vi "TesterOption (SubVI).vi"(8 "error in (no error)":errorcluster, 9 "On/Off":bool=TRUE, 10 "Tester Option":T1(ring), 11 "VISA Refnum in":refnum<visa-resource-name>) -> (0 "error out":errorcluster, 3 "VISA Refnum out":refnum<visa-resource-name>)   [LabVIEW 2017]
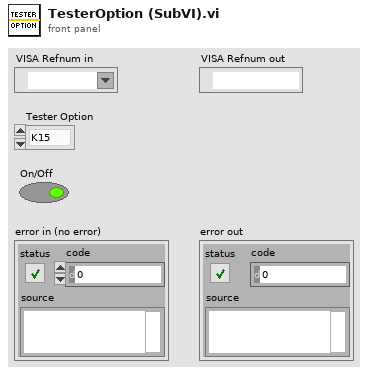
[diagram p1: front panel]
types:
  T1 = enum16{"K15", "K16", "K17", "Venable", "Firmeware", "Fan", "Power", "120C", "110C", "100C", "90C", "80C", "70C", "60C", "50C", "40C", "30C", "25C", "20C", "10C", "0C"}
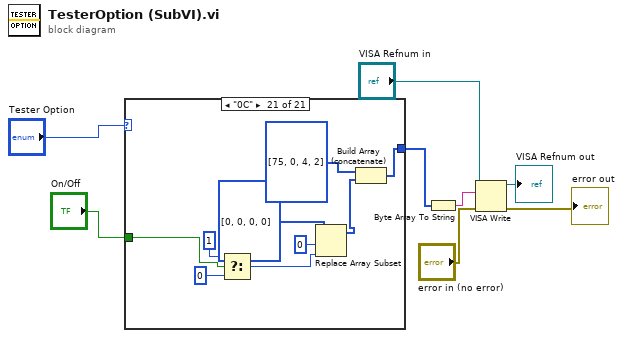
[diagram p0: block diagram]
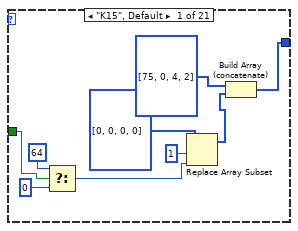
[diagram p2: hidden frame]
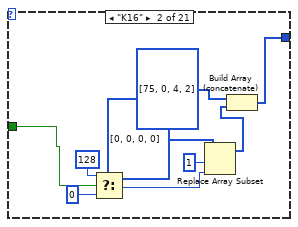
[diagram p3: hidden frame]
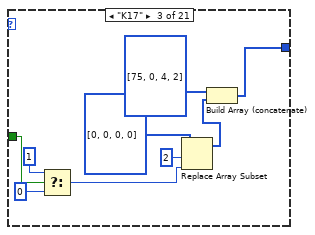
[diagram p4: hidden frame]
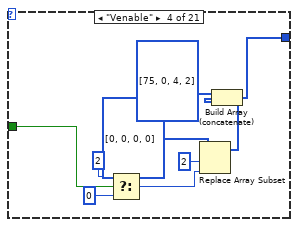
[diagram p5: hidden frame]
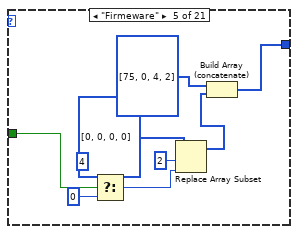
[diagram p6: hidden frame]
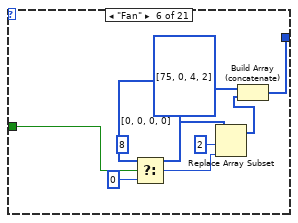
[diagram p7: hidden frame]
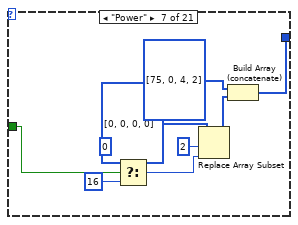
[diagram p8: hidden frame]
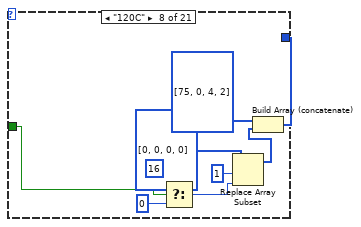
[diagram p9: hidden frame]
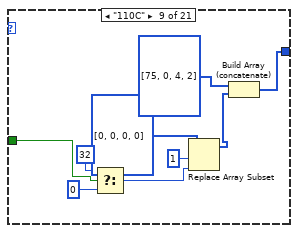
[diagram p10: hidden frame]
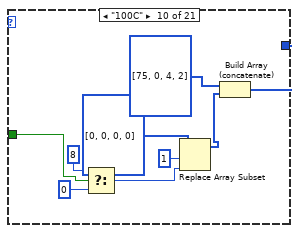
[diagram p11: hidden frame]
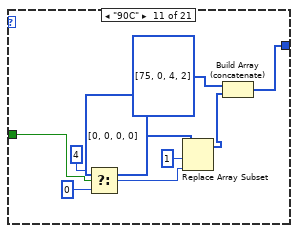
[diagram p12: hidden frame]
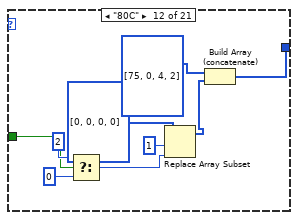
[diagram p13: hidden frame]
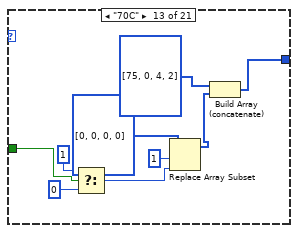
[diagram p14: hidden frame]
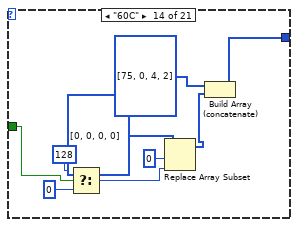
[diagram p15: hidden frame]
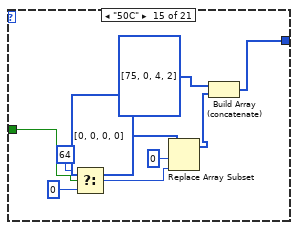
[diagram p16: hidden frame]
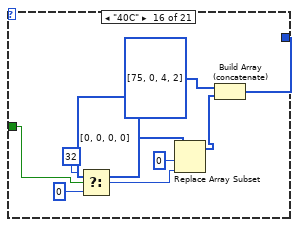
[diagram p17: hidden frame]
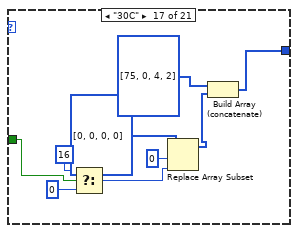
[diagram p18: hidden frame]
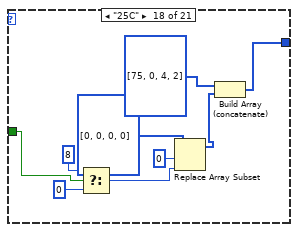
[diagram p19: hidden frame]
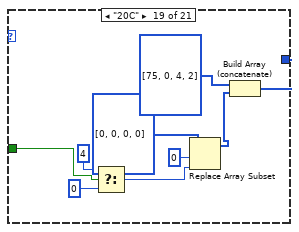
[diagram p20: hidden frame]
diagram:
  n1 = case shown="\"0C\"" "Tester Option" {
    tunnel: [w16 w25 w27 w43 w52 w61 w69 w72 w82 w91 w100 w109 w117 w127 w136 w145 w154 w163 w172 w181 w190] -> w4
    tunnel: "On/Off" -> [w10 w19 w28 w37 w46 w55 w65 w73 w81 w90 w99 w108 w118 w126 w135 w144 w153 w162 w171 w180 w189]
    frame "K15", Default {
      n2 = Select(t=u8 64, s=w10, f=u8 0) -> (s? t:f=w11:u8)
      n3 = Replace Array Subset(array=u8[] [0, 0, 0, 0], new element=w11, index=1) -> (w9:u8[])
      n4 = Build Array (concatenate)(u8[] [75, 0, 4, 2], w9) -> (w16:u8[])
    }
    frame "K16" {
      n5 = Select(t=u8 128, s=w19, f=u8 0) -> (s? t:f=w20:u8)
      n6 = Replace Array Subset(array=u8[] [0, 0, 0, 0], new element=w20, index=1) -> (w18:u8[])
      n7 = Build Array (concatenate)(u8[] [75, 0, 4, 2], w18) -> (w25:u8[])
    }
    frame "K17" {
      n8 = Select(t=u8 1, s=w28, f=u8 0) -> (s? t:f=w30:u8)
      n9 = Replace Array Subset(array=u8[] [0, 0, 0, 0], new element=w30, index=2) -> (w29:u8[])
      n10 = Build Array (concatenate)(u8[] [75, 0, 4, 2], w29) -> (w27:u8[])
    }
    frame "Venable" {
      n11 = Select(t=u8 2, s=w37, f=u8 0) -> (s? t:f=w38:u8)
      n12 = Replace Array Subset(array=u8[] [0, 0, 0, 0], new element=w38, index=2) -> (w36:u8[])
      n13 = Build Array (concatenate)(u8[] [75, 0, 4, 2], w36) -> (w43:u8[])
    }
    frame "Firmeware" {
      n14 = Select(t=u8 4, s=w46, f=u8 0) -> (s? t:f=w47:u8)
      n15 = Replace Array Subset(array=u8[] [0, 0, 0, 0], new element=w47, index=2) -> (w45:u8[])
      n16 = Build Array (concatenate)(u8[] [75, 0, 4, 2], w45) -> (w52:u8[])
    }
    frame "Fan" {
      n17 = Select(t=u8 8, s=w55, f=u8 0) -> (s? t:f=w56:u8)
      n18 = Replace Array Subset(array=u8[] [0, 0, 0, 0], new element=w56, index=2) -> (w54:u8[])
      n19 = Build Array (concatenate)(u8[] [75, 0, 4, 2], w54) -> (w61:u8[])
    }
    frame "Power" {
      n20 = Select(t=u8 0, s=w65, f=u8 16) -> (s? t:f=w63:u8)
      n21 = Replace Array Subset(array=u8[] [0, 0, 0, 0], new element=w63, index=2) -> (w68:u8[])
      n22 = Build Array (concatenate)(u8[] [75, 0, 4, 2], w68) -> (w69:u8[])
    }
    frame "120C" {
      n23 = Select(t=u8 16, s=w73, f=u8 0) -> (s? t:f=w75:u8)
      n24 = Replace Array Subset(array=u8[] [0, 0, 0, 0], new element=w75, index=1) -> (w74:u8[])
      n25 = Build Array (concatenate)(u8[] [75, 0, 4, 2], w74) -> (w72:u8[])
    }
    frame "110C" {
      n26 = Select(t=u8 32, s=w81, f=u8 0) -> (s? t:f=w84:u8)
      n27 = Replace Array Subset(array=u8[] [0, 0, 0, 0], new element=w84, index=1) -> (w83:u8[])
      n28 = Build Array (concatenate)(u8[] [75, 0, 4, 2], w83) -> (w82:u8[])
    }
    frame "100C" {
      n29 = Select(t=u8 8, s=w90, f=u8 0) -> (s? t:f=w93:u8)
      n30 = Replace Array Subset(array=u8[] [0, 0, 0, 0], new element=w93, index=1) -> (w92:u8[])
      n31 = Build Array (concatenate)(u8[] [75, 0, 4, 2], w92) -> (w91:u8[])
    }
    frame "90C" {
      n32 = Select(t=u8 4, s=w99, f=u8 0) -> (s? t:f=w102:u8)
      n33 = Replace Array Subset(array=u8[] [0, 0, 0, 0], new element=w102, index=1) -> (w101:u8[])
      n34 = Build Array (concatenate)(u8[] [75, 0, 4, 2], w101) -> (w100:u8[])
    }
    frame "80C" {
      n35 = Select(t=u8 2, s=w108, f=u8 0) -> (s? t:f=w111:u8)
      n36 = Replace Array Subset(array=u8[] [0, 0, 0, 0], new element=w111, index=1) -> (w110:u8[])
      n37 = Build Array (concatenate)(u8[] [75, 0, 4, 2], w110) -> (w109:u8[])
    }
    frame "70C" {
      n38 = Select(t=u8 1, s=w118, f=u8 0) -> (s? t:f=w120:u8)
      n39 = Replace Array Subset(array=u8[] [0, 0, 0, 0], new element=w120, index=1) -> (w119:u8[])
      n40 = Build Array (concatenate)(u8[] [75, 0, 4, 2], w119) -> (w117:u8[])
    }
    frame "60C" {
      n41 = Select(t=u8 128, s=w126, f=u8 0) -> (s? t:f=w129:u8)
      n42 = Replace Array Subset(array=u8[] [0, 0, 0, 0], new element=w129, index=0) -> (w128:u8[])
      n43 = Build Array (concatenate)(u8[] [75, 0, 4, 2], w128) -> (w127:u8[])
    }
    frame "50C" {
      n44 = Select(t=u8 64, s=w135, f=u8 0) -> (s? t:f=w138:u8)
      n45 = Replace Array Subset(array=u8[] [0, 0, 0, 0], new element=w138, index=0) -> (w137:u8[])
      n46 = Build Array (concatenate)(u8[] [75, 0, 4, 2], w137) -> (w136:u8[])
    }
    frame "40C" {
      n47 = Select(t=u8 32, s=w144, f=u8 0) -> (s? t:f=w147:u8)
      n48 = Replace Array Subset(array=u8[] [0, 0, 0, 0], new element=w147, index=0) -> (w146:u8[])
      n49 = Build Array (concatenate)(u8[] [75, 0, 4, 2], w146) -> (w145:u8[])
    }
    frame "30C" {
      n50 = Select(t=u8 16, s=w153, f=u8 0) -> (s? t:f=w156:u8)
      n51 = Replace Array Subset(array=u8[] [0, 0, 0, 0], new element=w156, index=0) -> (w155:u8[])
      n52 = Build Array (concatenate)(u8[] [75, 0, 4, 2], w155) -> (w154:u8[])
    }
    frame "25C" {
      n53 = Select(t=u8 8, s=w162, f=u8 0) -> (s? t:f=w165:u8)
      n54 = Replace Array Subset(array=u8[] [0, 0, 0, 0], new element=w165, index=0) -> (w164:u8[])
      n55 = Build Array (concatenate)(u8[] [75, 0, 4, 2], w164) -> (w163:u8[])
    }
    frame "20C" {
      n56 = Select(t=u8 4, s=w171, f=u8 0) -> (s? t:f=w174:u8)
      n57 = Replace Array Subset(array=u8[] [0, 0, 0, 0], new element=w174, index=0) -> (w173:u8[])
      n58 = Build Array (concatenate)(u8[] [75, 0, 4, 2], w173) -> (w172:u8[])
    }
    frame "10C" {
      n59 = Select(t=u8 2, s=w180, f=u8 0) -> (s? t:f=w183:u8)
      n60 = Replace Array Subset(array=u8[] [0, 0, 0, 0], new element=w183, index=0) -> (w182:u8[])
      n61 = Build Array (concatenate)(u8[] [75, 0, 4, 2], w182) -> (w181:u8[])
    }
    frame "0C" {
      n62 = Select(t=u8 1, s=w189, f=u8 0) -> (s? t:f=w192:u8)
      n63 = Replace Array Subset(array=u8[] [0, 0, 0, 0], new element=w192, index=0) -> (w191:u8[])
      n64 = Build Array (concatenate)(u8[] [75, 0, 4, 2], w191) -> (w190:u8[])
    }
  }
  n65 = Byte Array To String(unsigned byte array=w4) -> (string=w3:string)
  n66 = VISA Write(VISA resource name="VISA Refnum in", write buffer=w3, error in (no error)="error in (no error)") -> (VISA resource name out=→"VISA Refnum out":refnum<visa-resource-name>, error out=→"error out":errorcluster)  [unwired: 1 out]
